vi "2 Optical Motion (Overlay Eyes).vi"() -> ()   [LabVIEW 2012]
doc: "This example shows how to use the Lucas Kanade Pyramid motion estimation VI to track features in a sequence of images in NI Vision. The VI reads the frames from an AVI file and tracks user specified features in the image from frame to frame."
uses:
  Controls/EyeOptionsCluster.ctl
  <vilib>/userdefined/High Color/IMAQdx.ctl
  <vilib>/vision/driver/NI_Vision_Acquisition_Software.lvlib
  <vilib>/vision/NI_Vision_Development_Module.lvlib
panel:
  in  "Feature Coordinates":cluster{"X position":sgl, "Y Position":sgl}={"X position"=157.7922, "Y Position"=150.9804} {"X position" scale=0.0..300.0; "Y Position" scale=0.0..300.0}
  in  "Eye Options":T1={"Eye Size"=1.0, "Overlay Eyes?"=TRUE, "Eye Tracking?"=TRUE} {"Eye Size" items=["Small"=0.5, "Medium"=1, "Large"=2]}
  in  "Select Points":bool caption="Click on the image and select the points to track. Press the <Ctrl> key while selecting  multiple points. Press the  \"Select Points\" button after  all points have been selected."
  out "Image":T2(plugin-control)
  in  "Stop":bool
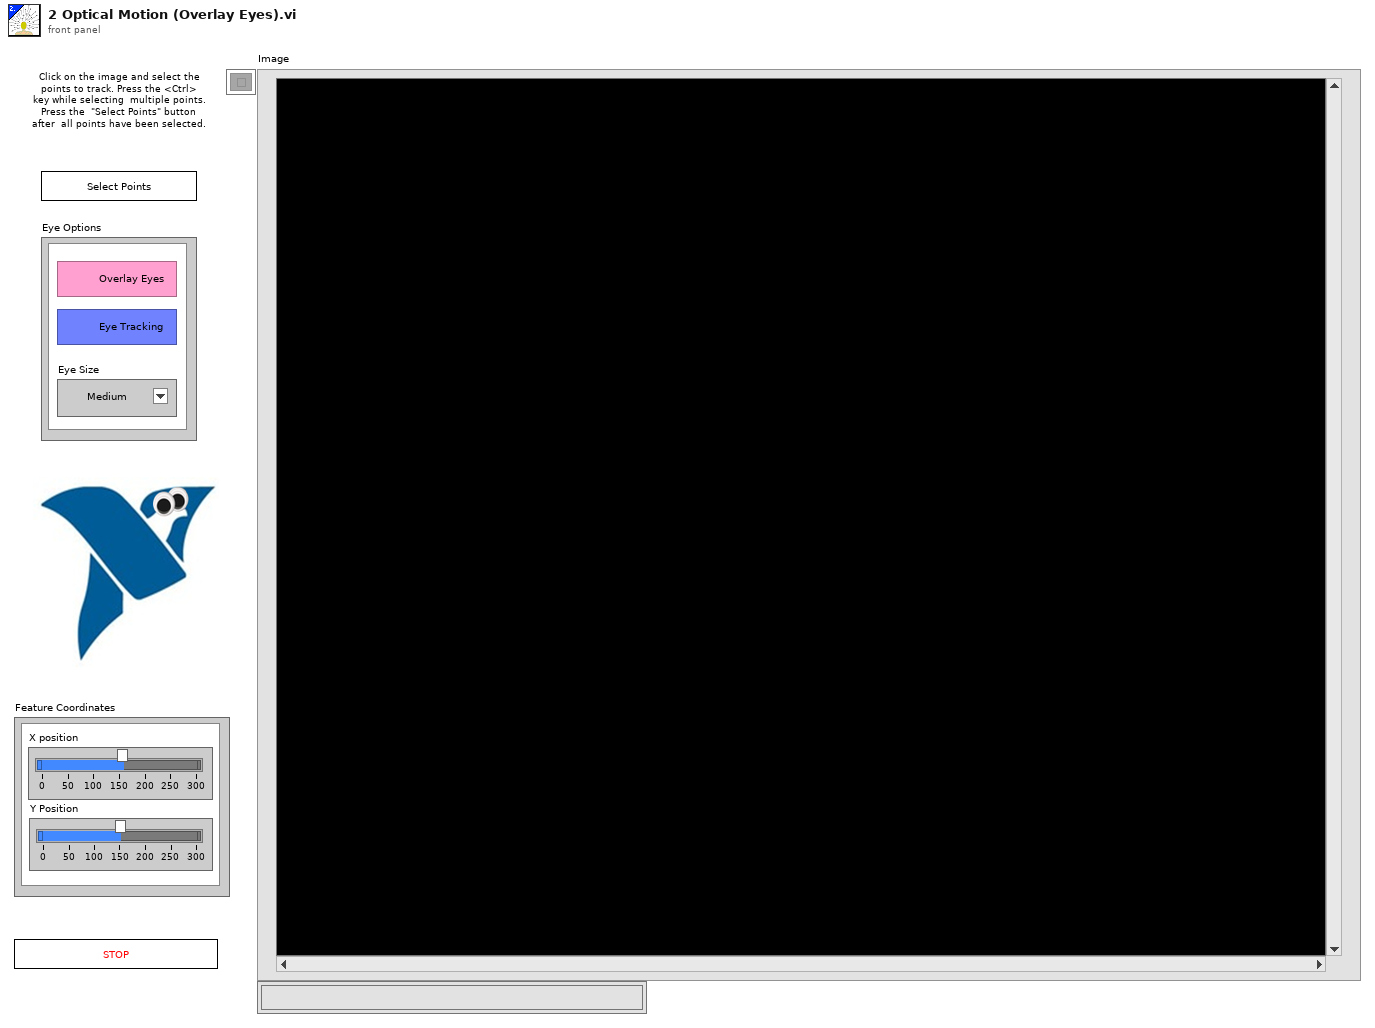
[diagram p1: front panel]
types:
  T1 = typedef "EyeOptionsCluster.ctl" = cluster{"Eye Size":sgl, "Overlay Eyes?":bool, "Eye Tracking?":bool}
  T2 = typedef "IMAQ Image.ctl" = refnum<image>
  T3 = typedef "IMAQdx.ctl" = refnum<k21>
  T4 = cluster{"Level":i32, "maxiteration":i32, "windowsize":i32, "threshold":dbl}
  T5 = cluster{"Global Rectangle":i32[], "Contours":cluster{"Contour Type":u32, "ROI Type":u32, "Points":i32[]}[]}
  T6 = typedef "ROI Descriptor" = cluster{"Global Rectangle":i32[], "Contours":cluster{"ID":enum32{"External", "Internal"}, "Type":u32, "Coordinates":i32[]}[]}
  T7 = typedef "IMAQ Point" = cluster{"X":sgl, "Y":sgl}
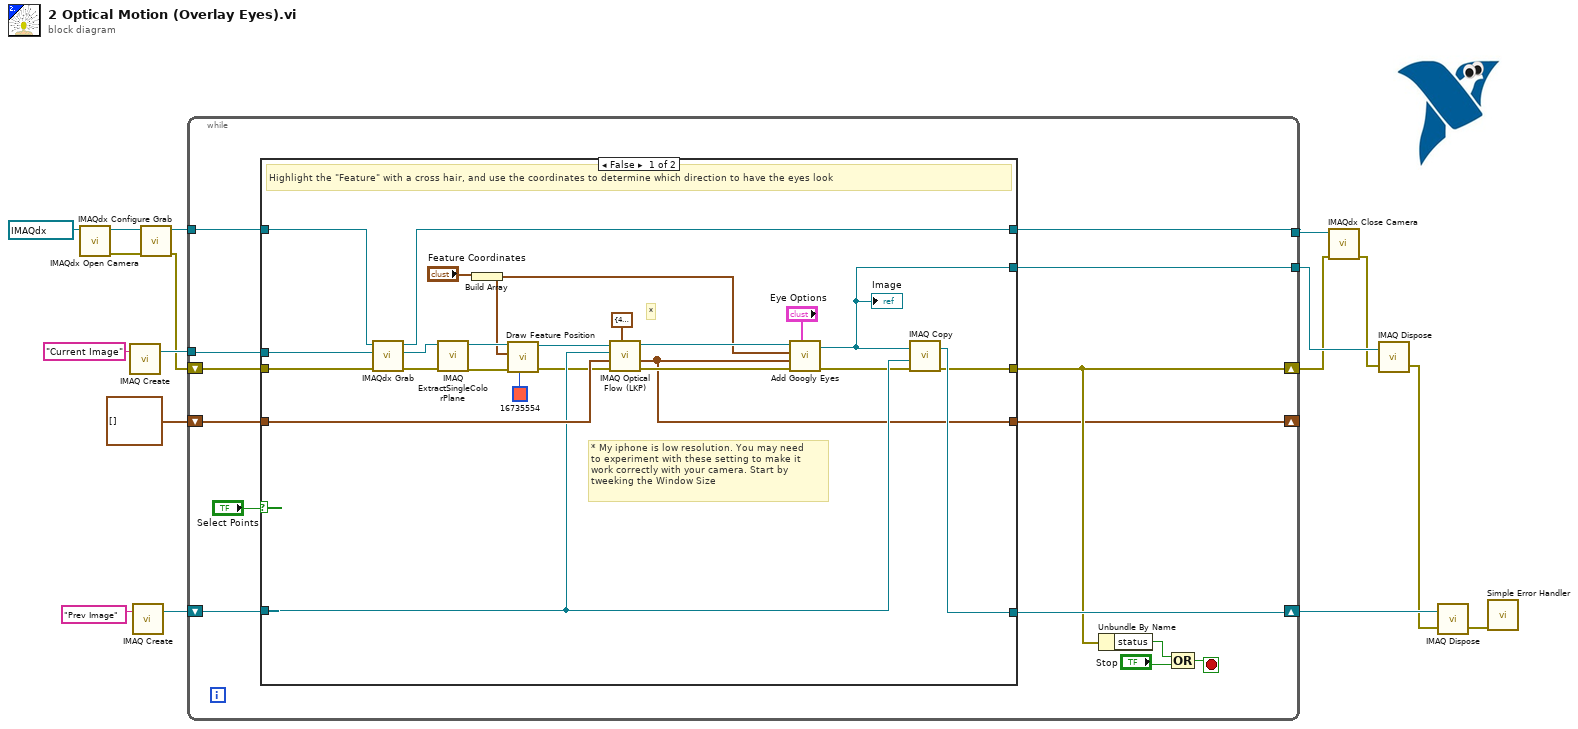
[diagram p0: block diagram]
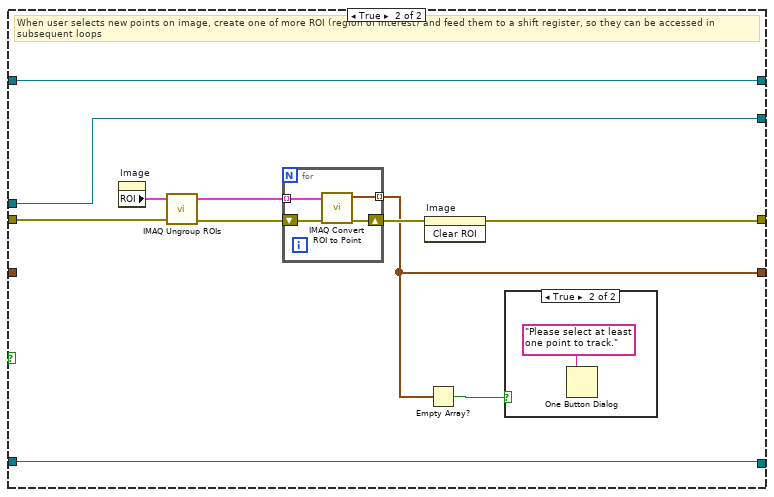
[diagram p2: hidden frame]
diagram:
  n1 = call <vilib>:"IMAQdx Open Camera.vi"("Session In"=T3 "iPhone") -> ("error out"=w9:errorcluster, "Session Out"=w10:T3)  [unwired: 9 in]
  n2 = call "IMAQ Create"("Image Name"="Current Image") -> ("New Image"=w16:T2)  [unwired: 3 in, 2 out]
  n3 = call "IMAQ Create"("Image Name"="Prev Image") -> ("New Image"=w1:T2)  [unwired: 3 in, 2 out]
  n4 = call <vilib>:"IMAQdx Configure Grab.vi"("error in"=w9, "Session In"=w10) -> ("error out"=w2:errorcluster, "Session Out"=w3:T3)  [unwired: 8 in]
  n5 = while {
    tunnel: w16 -> [w21]
    shift-right: [w26] -> w13
    shift-left: w1 -> [w28]
    shift-right: [w23] -> _
    shift-left: cluster{"X":sgl, "Y":sgl}[] [] ("Feature Points Out") -> [w24]
    shift-right: [w25] -> w7
    shift-left: w2 -> [w31]
    tunnel: [w20] -> w14
    tunnel: w3 -> [w19]
    tunnel: [w18] -> w12
    stop <- w29 stop-if-true
    n6 = case shown="False" "Select Points" {
      tunnel: w31 -> [w55 w61]
      tunnel: w21 -> [w54 w60]
      tunnel: w28 -> [w48 w66]
      tunnel: [w53 w66] -> w26
      tunnel: [w52 w57] -> w25
      tunnel: w24 -> [w51 _]
      tunnel: [w39 w59] -> w23
      tunnel: [w38 w60] -> w20
      tunnel: w19 -> [w50 w56]
      tunnel: [w49 w56] -> w18
      frame False {
        # "* My iphone is low resolution. You may need\nto experiment with these setting to make it\nwork correctly with your camera. Start by \ntweeking the Window Size"
        # "*"
        # "Highlight the \"Feature\" with a cross hair, and use the coordinates to determine which direction to have the eyes look"
        n7 = call <vilib>:"IMAQdx Grab.vi"("error in"=w55, "Image In"=w54, "Session In"=w50) -> ("error out"=w45:errorcluster, "Image Out"=w46:T2, "Session Out"=w49:T3)  [unwired: 5 in, 1 out]
        n8 = call "IMAQ ExtractSingleColorPlane"("error in (no error)"=w45, "Image Src"=w46) -> ("error out"=w36:errorcluster, "Image Dst Out"=w41:T2)  [unwired: 8 in]
        n9 = Build Array("Feature Coordinates") -> (w33:cluster{"X position":sgl, "Y Position":sgl}[])
        n10 = call "Draw Feature Position.vi"("Color"=u32 16735554, "Error In"=w36, "Feature Ponts"=w33, "Image"=w41) -> ("Error Out"=w32:errorcluster, "Image Out"=w40:T2)  [unwired: 6 in]
        n11 = call "IMAQ Optical Flow (LKP)"("Options"=T4 {"Level"=4, "maxiteration"=5, "windowsize"=15, "threshold"=0.01} ("Optical Flow Options"), "error in (no error)"=w32, "Feature Points In"=w51, "Previous Frame"=w48, "Current Frame"=w40) -> ("error out"=w44:errorcluster, "Feature Points Out"=w39:cluster{"X":sgl, "Y":sgl}[], "Current Frame Out (dup)"=w37:T2)  [unwired: 1 in, 3 out]
        n12 = call "Add Googly Eyes.vi"("Eye Options"="Eye Options", "error in (no error)"=w44, "Eye Coordinates"=w39, "Feature Coordinates"=w33, "ImageRef In"=w37) -> ("error out"=w47:errorcluster, "ImageRef out"=w38:T2)  [unwired: 5 in]
        "Image" <- w38
        n13 = call "IMAQ Copy"("error in (no error)"=w47, "Image Dst"=w48, "Image Src"=w38) -> ("error out"=w52:errorcluster, "Image Dst Out"=w53:T2)  [unwired: 3 out]
      }
      frame True {
        # "When user selects new points on image, create one of more ROI (region of interest) and feed them to a shift register, so they can be accessed in subsequent loops"
        n14 = property on="Image" class="ImageControl"() -> ("ROI"=w65:T5)  [unwired: 2 in, 2 out]
        n15 = call "IMAQ Ungroup ROIs"("error in (no error)"=w61, "ROI Descriptor"=w65) -> ("error out"=w64:errorcluster, "ROI Descriptors out"=w63:T6[])  [unwired: 2 out]
        n16 = for {
          shift-right: [w68] -> w62
          shift-left: w64 -> [w71]
          tunnel: w63 -> [w70] mode=indexing
          tunnel: [w69] -> w59 mode=indexing
          n17 = call "IMAQ Convert ROI to Point"("error in (no error)"=w71, "ROI Descriptor"=w70) -> ("error out"=w68:errorcluster, "Point"=w69:T7)  [unwired: 7 out]
        }
        n18 = invoke on="Image" class="ImageControl" method="Clear ROI"(error in=w62) -> (error out=w57:errorcluster)  [unwired: 2 in, 2 out]
        n19 = Empty Array?(array=w59) -> (empty?=w58:bool)
        n20 = case shown="True" w58 {
          frame False {
          }
          frame True {
            n21 = One Button Dialog(message="Please select at least one point to track.") -> ()  [unwired: 2 out]
          }
        }
      }
    }
    n22 = Unbundle By Name(w25) -> ("status"=w27:bool)
    n23 = Compound Arithmetic op=OR(w27, "Stop") -> (w29:bool)
  }
  n24 = call <vilib>:"IMAQdx Close Camera.vi"("error in"=w7, "Session In"=w12) -> ("error out"=w6:errorcluster)  [unwired: 9 in]
  n25 = call "IMAQ Dispose"("Image"=w14, "error in (no error)"=w6) -> ("error out"=w5:errorcluster)  [unwired: 1 in, 3 out]
  n26 = call "IMAQ Dispose"("Image"=w13, "error in (no error)"=w5) -> ("error out"=w4:errorcluster)  [unwired: 1 in, 3 out]
  n27 = call <vilib>:"Simple Error Handler.vi"("error in (no error)"=w4) -> ()  [unwired: 1 in, 8 out]
